vi "BigPowMod.vi"(1 "c":cluster{"Boolean":bool, "Array":u64[]}, 2 "b":cluster{"Boolean":bool, "Array":u64[]}, 3 "a":cluster{"Boolean":bool, "Array":u64[]}) -> (0 "a ^ b mod c":cluster{"Boolean":bool, "Array":u64[]})   [LabVIEW 2023]
panel:
  out "Numeric":i32
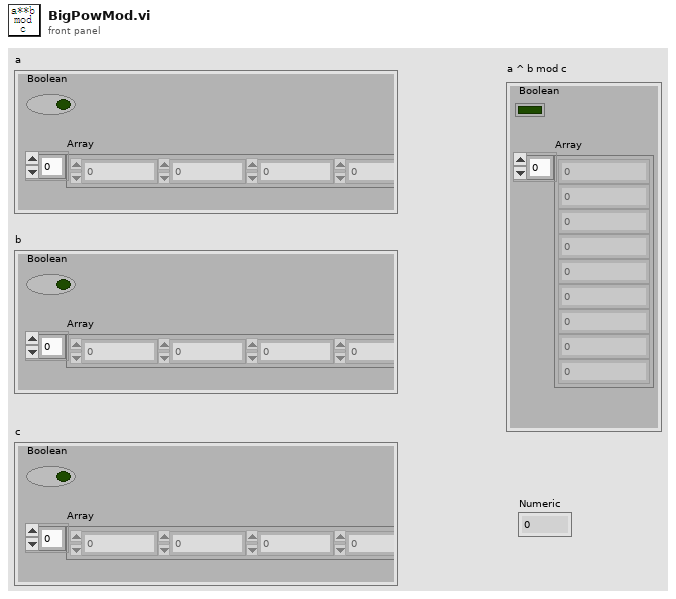
[diagram p1: front panel]
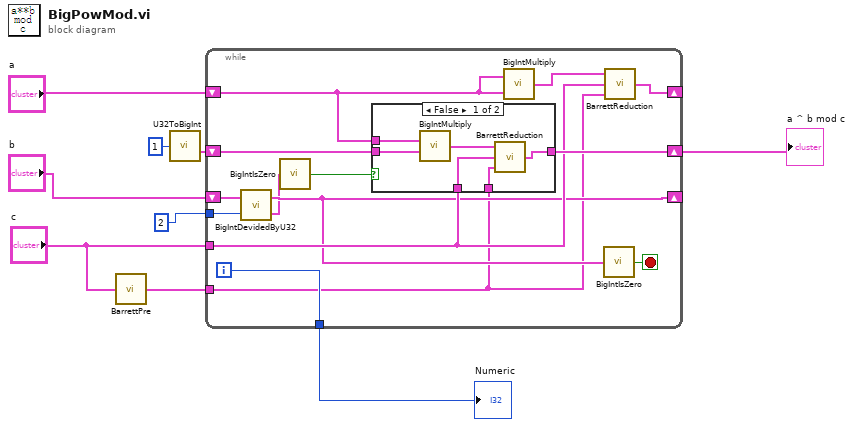
[diagram p0: block diagram]
diagram:
  n1 = call "BarrettPre.vi"("a"="c") -> ("mu"=w2:cluster{"Boolean":bool, "Array":u64[]})
  n2 = call "U32ToBigInt.vi"("U32 (<1e9)"=u32 1) -> ("Big Number"=w7:cluster{"P/N":bool, "Array":dbl[]})
  n3 = while {
    shift-right: [w15] -> _
    shift-left: "b" -> [w23]
    shift-right: [w17] -> _
    shift-left: "a" -> [w20]
    shift-right: [w21] -> w5
    shift-left: w7 -> [w22]
    tunnel: "c" -> [w18]
    tunnel: [w14] -> w4
    tunnel: w2 -> [w13]
    tunnel: u64 2 -> [w11]
    i -> [w14]
    stop <- w16 stop-if-true
    n4 = call "BigIntDevidedByU32.vi"("b (<1e9)"=w11, "a"=w23) -> ("a % b"=w12:cluster{"Boolean":bool, "Array":u64[]}, "a / b"=w15:cluster{"Boolean":bool, "Array":u64[]})
    n5 = call "BigIntIsZero.vi"("a"=w12) -> ("a = 0"=w10:bool)
    n6 = case shown="False" w10 {
      tunnel: w20 -> [w28 _]
      tunnel: w22 -> [w27 w30]
      tunnel: w18 -> [w26 _]
      tunnel: [w25 w30] -> w21
      tunnel: w13 -> [w24 _]
      frame False {
        n7 = call "BigIntMultiply.vi"("b"=w27, "a"=w28) -> ("a * b"=w29:cluster{"Boolean":bool, "Array":u64[]})
        n8 = call "BarrettReduction.vi"("mu"=w24, "b"=w26, "a"=w29) -> ("a % b"=w25:cluster{"Boolean":bool, "Array":u64[]})
      }
      frame True {
      }
    }
    n9 = call "BigIntMultiply.vi"("b"=w20, "a"=w20) -> ("a * b"=w19:cluster{"Boolean":bool, "Array":u64[]})
    n10 = call "BigIntIsZero.vi"("a"=w15) -> ("a = 0"=w16:bool)
    n11 = call "BarrettReduction.vi"("mu"=w13, "b"=w18, "a"=w19) -> ("a % b"=w17:cluster{"Boolean":bool, "Array":u64[]})
  }
  "a ^ b mod c" <- w5
  "Numeric" <- w4
